vi "Modbus Slave Example.vi"() -> ()   [LabVIEW 2013, in "Modbus Library - Advance.lvlib"]
doc: "An example of the modbus master functionality."
uses:
  Modbus Library - Advance.lvlib
  API/Wrapper/API Main.lvlib
  API/Slave/Modbus Slave.lvclass
  Data Model/Identification Parameters.ctl
  Data Model/Device Data Model.lvclass
  API/Wrapper/Create TCP Slave.vi
  Network Protocol/Network Slave/daemon status.ctl
  Network Protocol/Network Slave/Network Slave.lvclass
  Network Protocol/Network Slave/TCP/Connection.ctl
  Network Protocol/Network Slave/TCP/TCP Slave.lvclass
panel:
  in  "unit ID":u8=1
  out "TCP Connection List":T1[](array[typedef])
  out "TCP Connection Count":u32
  out "Daemon Error":errorcluster
  out "Daemon Status":T2
  in  "Stop Button":bool
  in  "Port":u16=502
  in  "Fetch Holding Registers":bool
  in  "Fetch Coils":bool
  in  "Set Discrete Inputs":bool
  in  "Set Input Registers":bool
  in  "Set Basic Objects":bool
  in  "Basic Objects":string[](array[string])=["National Instruments", "42", "1.0.0"]
  out "Status":string
  out "Holding Registers":u16[](array[numeric])
  in  "Input Registers":u16[](array[numeric])=[0, 0, 0, 0, 0, 0, 0, 0]
  out "Coils":bool[](array[boolean])
  in  "Discrete Inputs":bool[](array[boolean])
  # "Holding Registers are the integer outputs of a modbus device. This example allows you to read the first 8 outputs."
  # "Coils are the boolean outputs of a modbus device. This example allows you to read the first 8 outputs."
  # "Modbus devices can also store objects in their memory, which are variable length strings. This example sets the basic level of objects."
  # "Discrete inputs are the boolean inputs of a modbus device. This example allows you to set the first 8 inputs."
  # "Input Registers are the integer inputs of a modbus device. This example allows you to set the first 8 inputs."
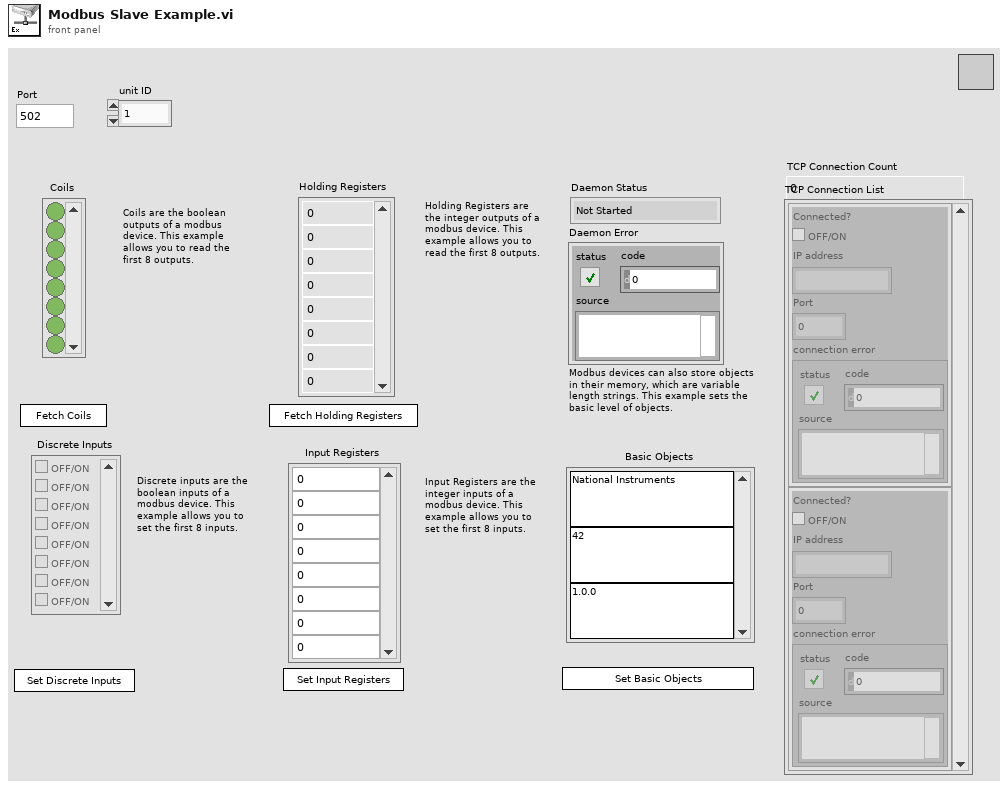
[diagram p1: front panel]
types:
  T1 = typedef "Modbus Library - Advance.lvlib/TCP Slave.lvclass/Connection.ctl" = cluster{"Connected?":bool, "IP address":string, "Port":u16, "connection error":errorcluster}
  T2 = typedef "Modbus Library - Advance.lvlib/Network Slave.lvclass/daemon status.ctl" = enum16{"Not Started", "Running", "Error", "Stopped"}
  T3 = typedef "Modbus Library - Advance.lvlib/Device Data Model.lvclass/Identification Parameters.ctl" = cluster{"Object ID":u8, "Value":string}
  T4 = typedef "Network Slave.lvclass/daemon status.ctl" = enum16{"Not Started", "Running", "Error", "Stopped"}
  T5 = typedef "K2Labs Modbus Library.lvlib/TCP Slave.lvclass/Connection.ctl" = cluster{"Connected?":bool, "IP address":string, "Port":u16, "connection error":errorcluster}
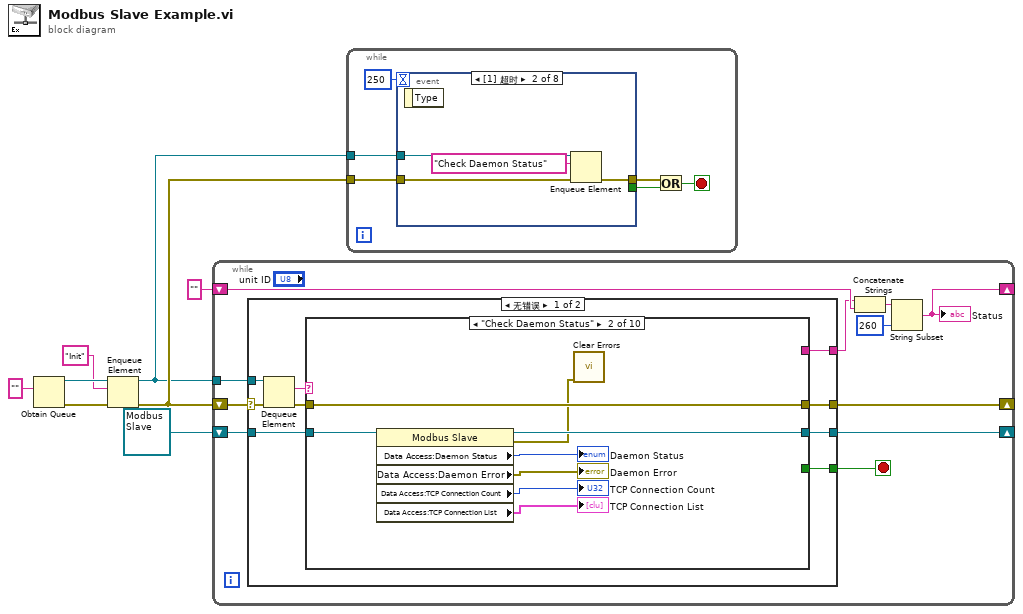
[diagram p0: block diagram]
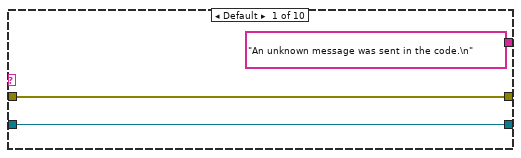
[diagram p2: hidden frame]
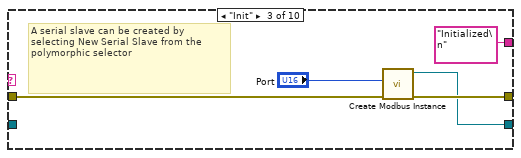
[diagram p3: hidden frame]
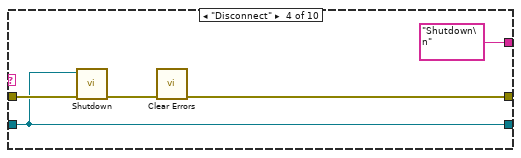
[diagram p4: hidden frame]
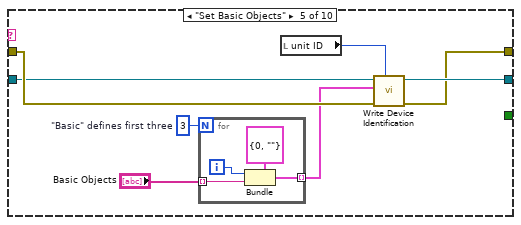
[diagram p5: hidden frame]
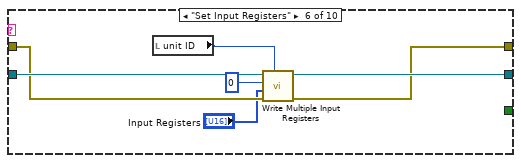
[diagram p6: hidden frame]
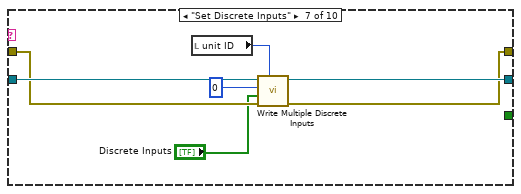
[diagram p7: hidden frame]
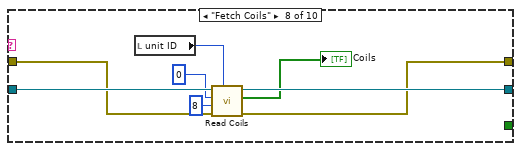
[diagram p8: hidden frame]
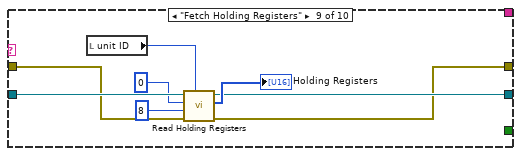
[diagram p9: hidden frame]
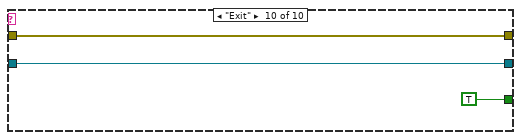
[diagram p10: hidden frame]
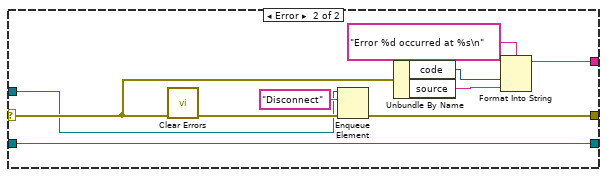
[diagram p11: hidden frame]
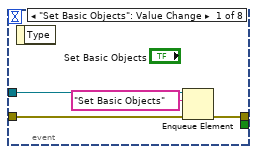
[diagram p12: hidden frame]
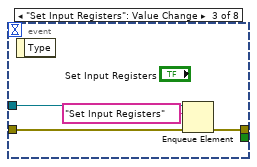
[diagram p13: hidden frame]
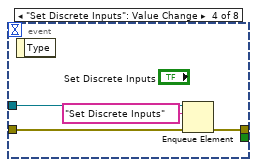
[diagram p14: hidden frame]
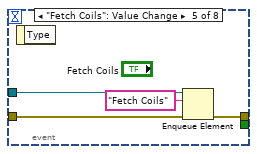
[diagram p15: hidden frame]
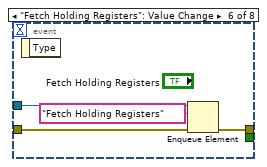
[diagram p16: hidden frame]
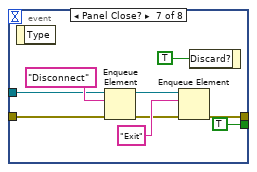
[diagram p17: hidden frame]
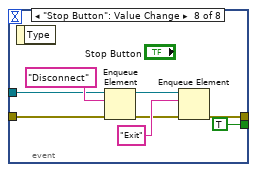
[diagram p18: hidden frame]
diagram:
  n1 = Obtain Queue(element data type="") -> (queue out=w4:refnum<queue>, error out=w8:errorcluster)  [unwired: 4 in, 1 out]
  n2 = Enqueue Element(queue=w4, element="Init", error in (no error)=w8) -> (queue out=w3:refnum<queue>, error out=w5:errorcluster)  [unwired: 1 in, 1 out]
  n3 = while {
    shift-right: [w9] -> _
    shift-left: refnum<class "Modbus Slave.lvclass"> refnum ("Modbus Slave") -> [w12]
    tunnel: w3 -> [w19]
    shift-right: [w10] -> _
    shift-left: w5 -> [w18]
    shift-right: [w17] -> _
    shift-left: "" ("Status") -> [w14]
    stop <- w11 stop-if-true
    n4 = case shown="无错误" w18 {
      selector: w18 -> [w27 w102]
      tunnel: w19 -> [w28 w96]
      tunnel: [w24 w103] -> w10
      tunnel: [w21 w99] -> w13
      tunnel: [w23 w95] -> w9
      tunnel: w12 -> [w22 w95]
      tunnel: [w20 _] -> w11
      frame No Error {
        n5 = Dequeue Element(queue=w28, error in (no error)=w27) -> (element=w25:string, error out=w26:errorcluster)  [unwired: 1 in, 2 out]
        n6 = case shown="\"Check Daemon Status\"" w25 {
          tunnel: w26 -> [w31 w39 w44 w49 w57 w65 w72 w80 w90 w94]
          tunnel: [w31 w39 w43 w45 w52 w66 w73 w78 w87 w94] -> w24
          tunnel: [w30 w37 w42 w47 w56 w67 w74 w79 w88 w93] -> w23
          tunnel: w22 -> [w30 w38 _ w47 w55 w68 w75 w83 w91 w93]
          tunnel: ["An unknown message was sent in the code.\n" _ "Initialized\n" "Shutdown\n" _ _ _ _ _ _] -> w21
          tunnel: [_ _ _ _ _ _ _ _ _ TRUE] -> w20
          frame Default {
          }
          frame "Check Daemon Status" {
            n7 = property class="Modbus Slave"(reference=w38) -> (reference out=w37:refnum<class "Modbus Slave.lvclass">, error out=w36:errorcluster, "Data Access:Daemon Status"=→"Daemon Status":T4, "Data Access:Daemon Error"=→"Daemon Error":errorcluster, "Data Access:TCP Connection Count"=→"TCP Connection Count":u32, "Data Access:TCP Connection List"=→"TCP Connection List":T5[])  [unwired: 1 in]
            n8 = call <vilib>:"Clear Errors.vi"("error in (no error)"=w36) -> ()  [unwired: 6 in, 1 out]
          }
          frame "Init" {
            # "A serial slave can be created by selecting New Serial Slave from the polymorphic selector"
            n9 = call-poly "Create Modbus Instance.vi"("error in"=w44, "port (502)"="Port") -> ("error out"=w43:errorcluster, "TCP slave instance"=w42:refnum<class "Modbus Slave.lvclass">)  [unwired: 8 in]
          }
          frame "Disconnect" {
            n10 = call-dynamic "Shutdown.vi"("error in"=w49, "Modbus slave in"=w47) -> ("error out"=w48:errorcluster)  [unwired: 9 in]
            n11 = call <vilib>:"Clear Errors.vi"("error in (no error)"=w48) -> ("error out"=w45:errorcluster)  [unwired: 6 in]
          }
          frame "Set Basic Objects" {
            w51 = 3  # "Basic" defines first three
            n12 = for {
              N: w51 -> [_]
              tunnel: "Basic Objects" -> [w59] mode=indexing
              tunnel: [w58] -> w53 mode=indexing
              i -> [w60]
              n13 = Bundle(cluster=T3 {"Object ID"=0, "Value"=""} ("Parameters"), "Object ID"=w60, "Value"=w59) -> (w58:T3)
            }
            n14 = local read "unit ID"() -> (w50:u8)
            n15 = call-dynamic "Write Device Identification.vi"("unit ID"=w50, "error in"=w57, "objects"=w53, "Modbus slave in"=w55) -> ("error out"=w52:errorcluster, "Modbus slave out"=w56:refnum<class "Modbus Slave.lvclass">)  [unwired: 6 in]
          }
          frame "Set Input Registers" {
            n16 = local read "unit ID"() -> (w62:u8)
            n17 = call-dynamic "Write Multiple Input Registers.vi"("unit ID"=w62, "error in"=w65, "input registers to write"="Input Registers", "starting address"=u16 0, "Modbus slave in"=w68) -> ("error out"=w66:errorcluster, "Modbus slave out"=w67:refnum<class "Modbus Slave.lvclass">)  [unwired: 5 in]
          }
          frame "Set Discrete Inputs" {
            n18 = local read "unit ID"() -> (w69:u8)
            n19 = call-dynamic "Write Multiple Discrete Inputs.vi"("unit ID"=w69, "error in"=w72, "discrete inputs to write"="Discrete Inputs", "starting address"=u16 0, "Modbus slave in"=w75) -> ("error out"=w73:errorcluster, "Modbus slave out"=w74:refnum<class "Modbus Slave.lvclass">)  [unwired: 5 in]
          }
          frame "Fetch Coils" {
            n20 = local read "unit ID"() -> (w76:u8)
            n21 = call-dynamic "Read Coils.vi"("unit ID"=w76, "error in"=w80, "number of inputs"=u16 8 ("number of coils"), "starting address"=u16 0, "Modbus slave in"=w83) -> ("error out"=w78:errorcluster, "coils"=→"Coils":bool[], "Modbus slave out"=w79:refnum<class "Modbus Slave.lvclass">)  [unwired: 4 in]
          }
          frame "Fetch Holding Registers" {
            n22 = local read "unit ID"() -> (w84:u8)
            n23 = call-dynamic "Read Holding Registers.vi"("unit ID"=w84, "error in"=w90, "number of inputs"=u16 8 ("number of registers"), "starting address"=u16 0, "Modbus slave in"=w91) -> ("error out"=w87:errorcluster, "register values"=→"Holding Registers":u16[], "Modbus slave out"=w88:refnum<class "Modbus Slave.lvclass">)  [unwired: 4 in]
          }
          frame "Exit" {
          }
        }
      }
      frame Error {
        n24 = call <vilib>:"Clear Errors.vi"("error in (no error)"=w102) -> ("error out"=w104:errorcluster)  [unwired: 6 in]
        n25 = Enqueue Element(queue=w96, element="Disconnect", error in (no error)=w104) -> (error out=w103:errorcluster)  [unwired: 1 in, 2 out]
        n26 = Unbundle By Name(w102) -> ("code"=w101:i32, "source"=w100:string)
        n27 = Format Into String(format string="Error %d occurred at %s\n", w101, w100) -> (resulting string=w99:string)  [unwired: 2 in, 1 out]
      }
    }
    n28 = Concatenate Strings(w13, w14) -> (w15:string)
    n29 = String Subset(string=w15, length (rest)=260 ("length (rest)")) -> (substring=w17:string)  [unwired: 1 in]
    "Status" <- w17
  }
  n30 = while {
    tunnel: w5 -> [w110]
    tunnel: w3 -> [w109]
    stop <- w106 stop-if-true
    n31 = event shown="[1] 超时" {
      selector: _ -> [_ _ _ _ _ _ _ _]
      dyn-events: _ -> [_ _ _ _ _ _ _ _]
      timeout: 250 -> [_ _ _ _ _ _ _ _]
      tunnel: w110 -> [w114 w118 w122 w126 w130 w134 w140 w149]
      tunnel: [w113 w117 w121 w125 w129 w133 w135 w144] -> w108
      tunnel: w109 -> [w112 w116 w120 w124 w128 w132 w137 w146]
      tunnel: [_ _ _ _ _ _ TRUE ("Discard?") TRUE ("Discard?")] -> w107
      event "Set Basic Objects": Value Change {
        n32 = event-data() -> ()  [unwired: 1 in, 1 out]
        n33 = Enqueue Element(queue=w112, element="Set Basic Objects", error in (no error)=w114) -> (error out=w113:errorcluster)  [unwired: 1 in, 2 out]
      }
      event Timeout {
        n34 = event-data() -> ()  [unwired: 1 in, 1 out]
        n35 = Enqueue Element(queue=w116, element="Check Daemon Status", error in (no error)=w118) -> (error out=w117:errorcluster)  [unwired: 1 in, 2 out]
      }
      event "Set Input Registers": Value Change {
        n36 = event-data() -> ()  [unwired: 1 in, 1 out]
        n37 = Enqueue Element(queue=w120, element="Set Input Registers", error in (no error)=w122) -> (error out=w121:errorcluster)  [unwired: 1 in, 2 out]
      }
      event "Set Discrete Inputs": Value Change {
        n38 = event-data() -> ()  [unwired: 1 in, 1 out]
        n39 = Enqueue Element(queue=w124, element="Set Discrete Inputs", error in (no error)=w126) -> (error out=w125:errorcluster)  [unwired: 1 in, 2 out]
      }
      event "Fetch Coils": Value Change {
        n40 = event-data() -> ()  [unwired: 1 in, 1 out]
        n41 = Enqueue Element(queue=w128, element="Fetch Coils", error in (no error)=w130) -> (error out=w129:errorcluster)  [unwired: 1 in, 2 out]
      }
      event "Fetch Holding Registers": Value Change {
        n42 = event-data() -> ()  [unwired: 1 in, 1 out]
        n43 = Enqueue Element(queue=w132, element="Fetch Holding Registers", error in (no error)=w134) -> (error out=w133:errorcluster)  [unwired: 1 in, 2 out]
      }
      event Panel Close? {
        n44 = event-data() -> ()  [unwired: 1 in, 1 out]
        n45 = Enqueue Element(queue=w137, element="Disconnect", error in (no error)=w140) -> (queue out=w138:refnum<queue>, error out=w136:errorcluster)  [unwired: 1 in, 1 out]
        n46 = Enqueue Element(queue=w138, element="Exit", error in (no error)=w136) -> (error out=w135:errorcluster)  [unwired: 1 in, 2 out]
        n47 = event-data("Discard?"=TRUE) -> ()  [unwired: 1 in, 1 out]
      }
      event "Stop Button": Value Change {
        n48 = event-data() -> ()  [unwired: 1 in, 1 out]
        n49 = Enqueue Element(queue=w146, element="Disconnect", error in (no error)=w149) -> (queue out=w147:refnum<queue>, error out=w145:errorcluster)  [unwired: 1 in, 1 out]
        n50 = Enqueue Element(queue=w147, element="Exit", error in (no error)=w145) -> (error out=w144:errorcluster)  [unwired: 1 in, 2 out]
      }
    }
    n51 = Or(x=w108, y=w107) -> (x .or. y?=w106:bool)
  }
